vi "Braise.vi"(8 "error in (no error)":errorcluster, 11 "Appliance in":refnum<class "Appliance.lvclass">) -> (0 "error out":errorcluster, 3 "Appliance out":refnum<class "Appliance.lvclass">)   [LabVIEW 2020, in "Appliance.lvclass"]
uses:
  Appliance.lvclass
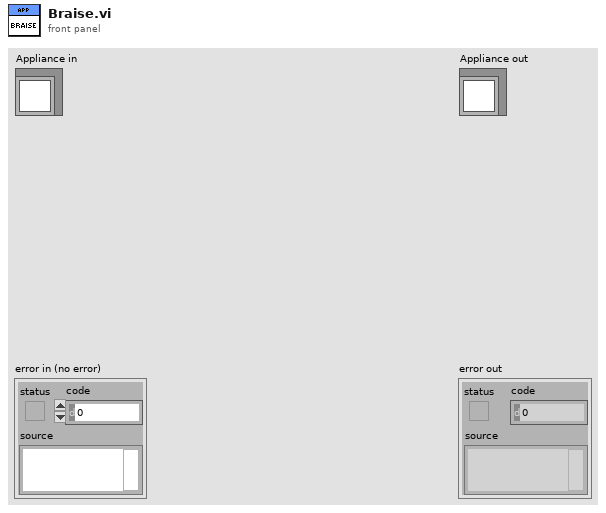
[diagram p1: front panel]
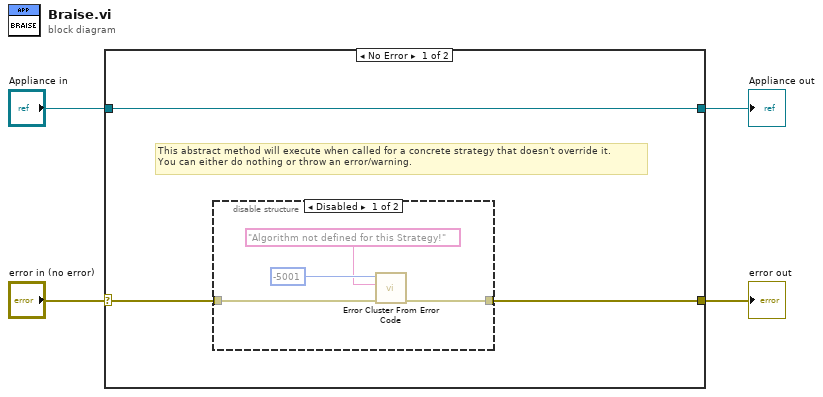
[diagram p0: block diagram]
diagram:
  n1 = case shown="No Error" "error in (no error)" {
    selector: "error in (no error)" -> [w6 w14]
    tunnel: [w5 w14] -> w1
    tunnel: [w7 w13] -> w3
    tunnel: "Appliance in" -> [w7 w13]
    frame No Error {
      # "This abstract method will execute when called for a concrete strategy that doesn't override it.\nYou can either do nothing or throw an error/warning."
      n2 = disable-structure shown="Disabled" {
        disable-tunnel: w6 -> [w11 w12]
        disable-tunnel: [w10 w12] -> w5
        frame Disabled {
          n3 = call <vilib>:"Error Cluster From Error Code.vi"("error in (no error)"=w11, "error message (\"\")"="Algorithm not defined for this Strategy!" ("error message (\"\")"), "error code (0)"=-5001) -> ("error out"=w10:errorcluster)  [unwired: 6 in]
        }
        frame Enabled {
        }
      }
    }
    frame Error {
    }
  }
  "error out" <- w1
  "Appliance out" <- w3
